vi "Init VacuumLine Config Obj by Label.vi"(8 "error in (no error)":errorcluster, 10 "label":string, 11 "VacuumLines Configuration in":refnum<class "VacuumLines Configuration.lvclass">) -> (0 "error out":errorcluster, 1 "not found?":bool, 2 "VacuumLine Configuration Obj":refnum<class "VacuumLine Configuration.lvclass">, 3 "VacuumLines Configuration out":refnum<class "VacuumLines Configuration.lvclass">)   [LabVIEW 2016, in "Hardware.lvlib" / "VacuumLine.lvlib" / "VacuumLines Configuration.lvclass"]
uses:
  <userlib>/Common Components/Hardware/Abstract System/VacuumLine/VacuumLines Configuration/VacuumLines Configuration.lvclass
  C:/Program Files (x86)/National Instruments/LabVIEW 2016/user.lib/Configuration Dialog Actor/Configuration.lvclass
  <userlib>/Common Components/Hardware/Abstract System/VacuumLine/VacuumLine Config/VacuumLine Configuration.lvclass
  <userlib>/Common Components/Hardware/Abstract System/VacuumLine/VacuumLines Configuration/VacuumLines Configuration.lvclass/VacuumLines Configuration.ctl
  <userlib>/Configuration Dialog Actor/Configuration.lvclass/Configuration.ctl
  <userlib>/Common Components/Hardware/Abstract System/VacuumLine/VacuumLines/VacuumLines.lvclass/VacuumLines.ctl
  <userlib>/Common Components/Hardware/Abstract System/VacuumLine/VacuumLine/VacuumLine.lvclass/VacuumLine.ctl
  <userlib>/Common Components/Hardware/Abstract System/VacuumLine/VacuumLine Config/VacuumLine Configuration.lvclass/VacuumLine Configuration.ctl
  <userlib>/Common Components/Hardware/Abstract System/VacuumLine/VacuumLine Config/Accessors/Write VacuumLine Obj.vi
  <userlib>/Configuration Dialog Actor/Accessors/Write Change Display.vi
  <userlib>/Configuration Dialog Actor/Accessors/Write Sub Panel.vi
  <userlib>/Configuration Dialog Actor/Accessors/Write Title.vi
  <userlib>/Configuration Dialog Actor/Accessors/Write Categories.vi
  <userlib>/Common Components/Hardware/Abstract System/VacuumLine/VacuumLine/Read Label.vi
  <userlib>/Common Components/Hardware/Abstract System/VacuumLine/VacuumLines Configuration/Accessors/Read VacuumLines Obj.vi
  <userlib>/Configuration Dialog Actor/Accessors/Read Change Display.vi
  <userlib>/Configuration Dialog Actor/Accessors/Read Sub Panel.vi
  <userlib>/Configuration Dialog Actor/Accessors/Read Title.vi
  <userlib>/Configuration Dialog Actor/Accessors/Read Categories.vi
  <userlib>/Common Components/Hardware/Abstract System/VacuumLine/VacuumLines/VacuumLines.lvclass
  <userlib>/Common Components/Hardware/Abstract System/VacuumLine/VacuumLine/VacuumLine.lvclass
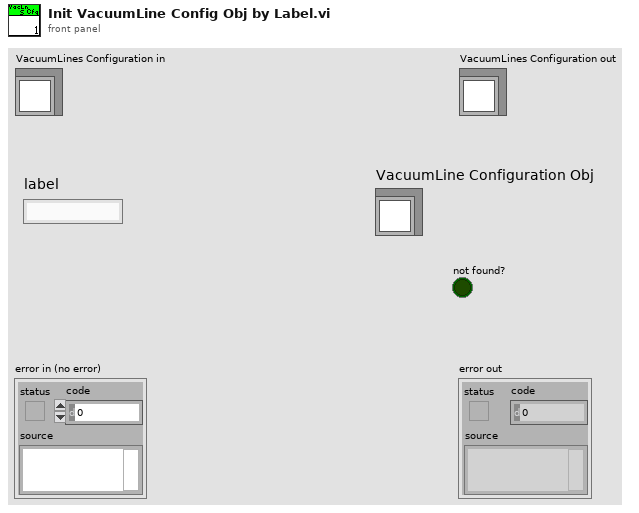
[diagram p1: front panel]
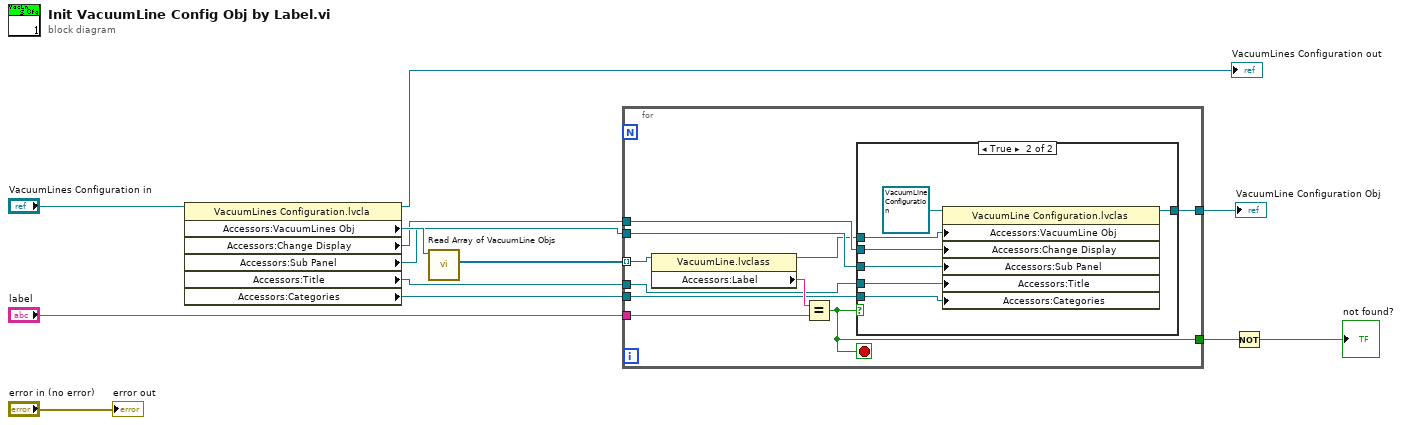
[diagram p0: block diagram]
diagram:
  n1 = property class="VacuumLines Configuration.lvcla"(reference="VacuumLines Configuration in") -> (reference out=→"VacuumLines Configuration out":refnum<class "VacuumLines Configuration.lvclass">, "Accessors:VacuumLines Obj"=w6:refnum<class "VacuumLines.lvclass">, "Accessors:Change Display"=w4:refnum<user-event>, "Accessors:Sub Panel"=w3:refnum<vi>, "Accessors:Title"=w2:refnum<vi>, "Accessors:Categories"=w1:refnum<vi>)  [unwired: 1 in, 1 out]
  n2 = call <userlib>:"Read Array of VacuumLine Objs.vi"("VacuumLines in"=w6) -> ("Array of VacuumLine Objs"=w8:refnum<class "VacuumLine.lvclass">[])  [unwired: 9 in, 1 out]
  n3 = for {
    tunnel: w8 -> [w23] mode=indexing
    tunnel: "label" -> [w21]
    tunnel: [w14] -> w11
    tunnel: [w20] -> w10
    tunnel: w4 -> [w19]
    tunnel: w3 -> [w18]
    tunnel: w2 -> [w17]
    tunnel: w1 -> [w16]
    stop <- w20 stop-if-true
    n4 = property class="VacuumLine.lvclass"(reference=w23) -> (reference out=w15:refnum<class "VacuumLine.lvclass">, "Accessors:Label"=w22:string)  [unwired: 1 in, 1 out]
    n5 = Equal?(x=w22, y=w21) -> (x = y?=w20:bool)
    n6 = case shown="True" w20 {
      tunnel: w19 -> [_ w28]
      tunnel: w18 -> [_ w27]
      tunnel: w17 -> [_ w26]
      tunnel: w16 -> [_ w25]
      tunnel: w15 -> [_ w24]
      tunnel: [_ w30] -> w14
      frame False {
      }
      frame True {
        n7 = property class="VacuumLine Configuration.lvclas"(reference=refnum<class "VacuumLine Configuration.lvclass"> refnum ("Hardware.lvlib:VacuumLine.lvlib:VacuumLine Configuration.lvclass"), "Accessors:VacuumLine Obj"=w24, "Accessors:Change Display"=w28, "Accessors:Sub Panel"=w27, "Accessors:Title"=w26, "Accessors:Categories"=w25) -> (reference out=w30:refnum<class "VacuumLine Configuration.lvclass">)  [unwired: 1 in, 1 out]
      }
    }
  }
  "VacuumLine Configuration Obj" <- w11
  n8 = Not(x=w10) -> (.not. x?=→"not found?":bool)
  "error out" <- "error in (no error)"
